vi "ADS-B.vi"() -> ()   [LabVIEW 2020, in "rtlsdr.lvlib"]
uses:
  rtlsdr.lvlib
panel:
  out "second subarray":u8[](array[numeric]) format="%08x"
  out "appended array 2":u8[][](array[numeric]) format="%08x"
  out "substring":string
  out "concatenated string":string
  out "Sample Buffer":u8[](array[numeric])
  in  "stop":bool
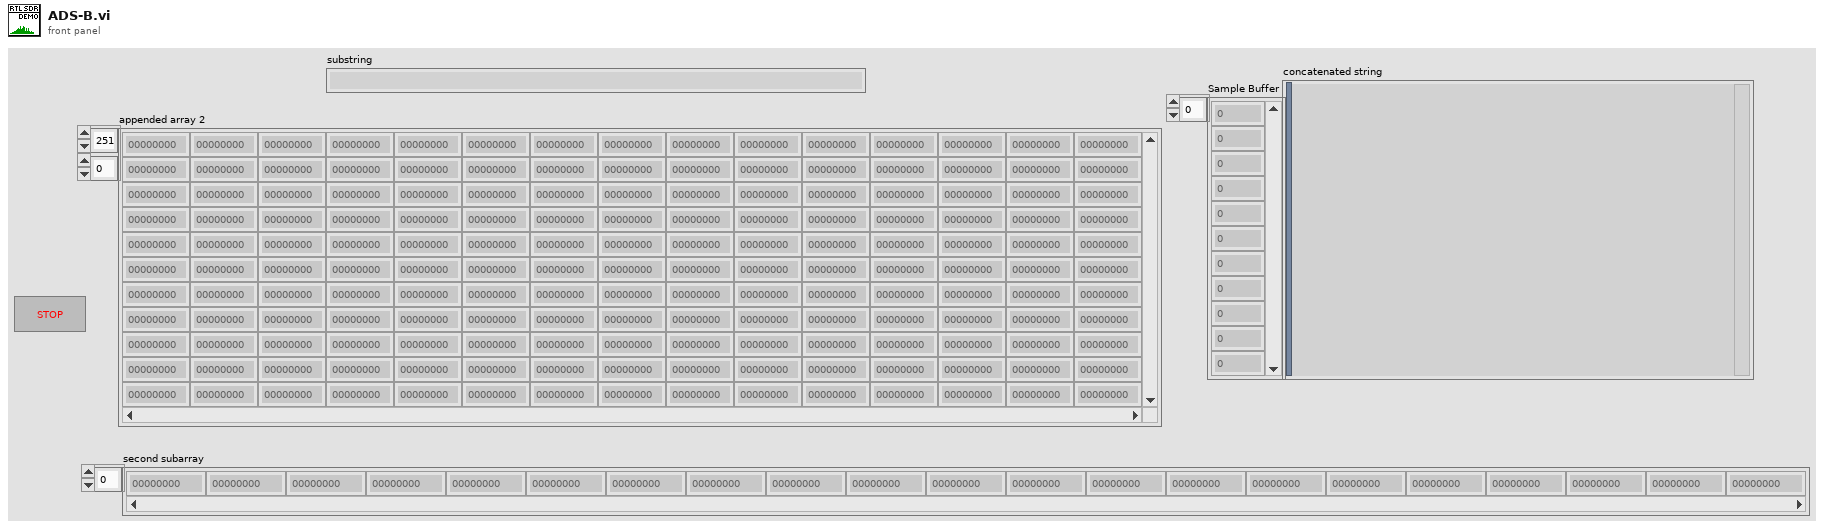
[diagram p1: front panel]
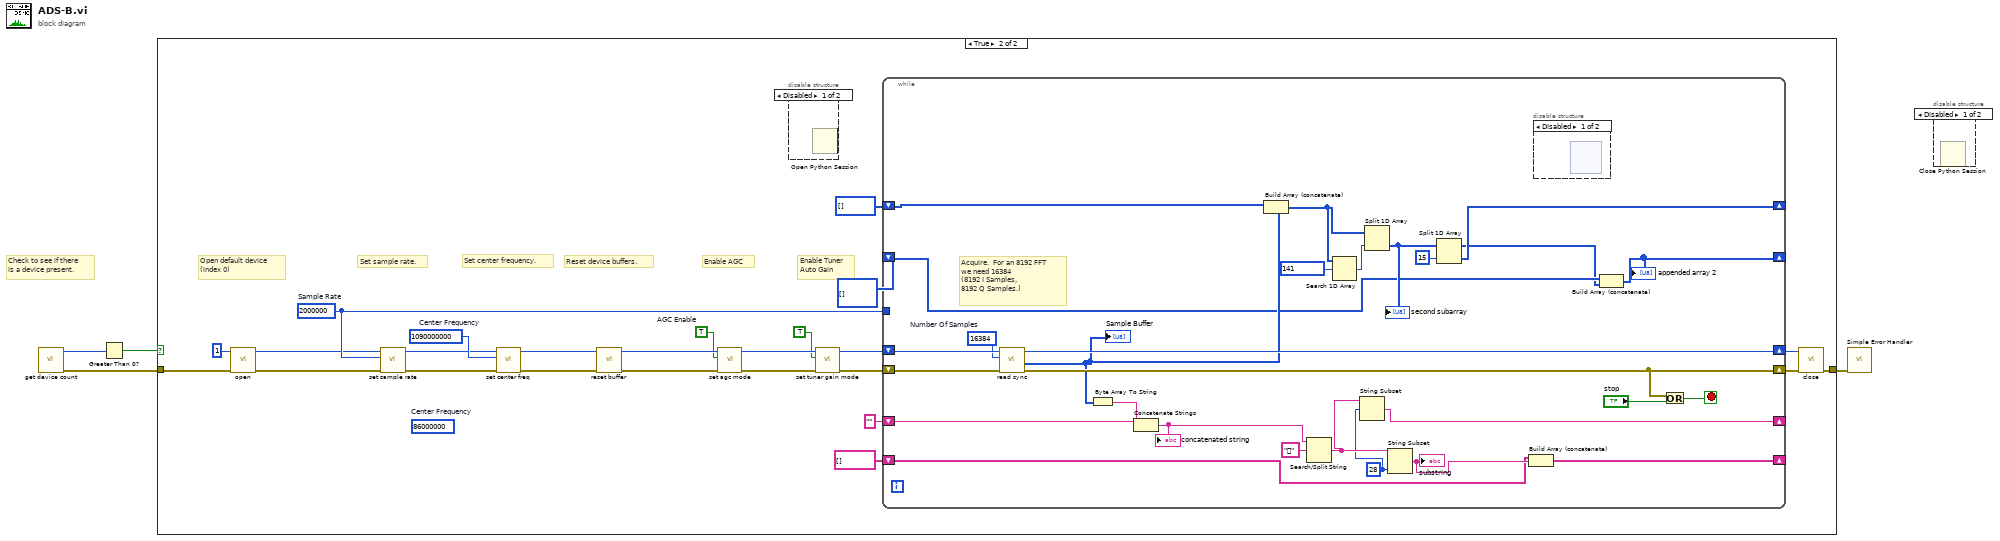
[diagram p0: block diagram]
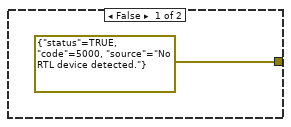
[diagram p3: hidden frame]
diagram:
  # "Check to see if there\nis a device present."
  n1 = call "get device count.vi"() -> ("error out"=w3:errorcluster, "Device Count"=w2:u32)  [unwired: 10 in]
  n2 = Greater Than 0?(x=w2) -> (x > 0?=w1:bool)
  n3 = case shown="True" w1 {
    tunnel: [errorcluster {"status"=TRUE, "code"=5000, "source"="No RTL device detected."} ("error out") w13] -> w4
    tunnel: w3 -> [_ w12]
    frame False {
    }
    frame True {
      (unwired) u32 86000000  # Center Frequency
      w16 = u32 1090000000  # Center Frequency
      w22 = TRUE  # AGC Enable
      w27 = u32 2000000  # Sample Rate
      # "Enable Tuner\nAuto Gain"
      # "Enable AGC"
      # "Reset device buffers."
      # "Set center frequency."
      # "Set sample rate."
      # "Open default device\n(index 0)"
      n4 = call "open.vi"("error in (no error)"=w12, "Device Index"=u32 1 ("index")) -> ("error out"=w17:errorcluster, "DeviceRefnum Out"=w18:u64)  [unwired: 6 in]
      n5 = call "set sample rate.vi"("error in (no error)"=w17, "Sample Rate"=w27, "DeviceRefnum"=w18) -> ("error out"=w15:errorcluster, "DeviceRefnum Out"=w14:u64)  [unwired: 6 in, 1 out]
      n6 = call "set center freq.vi"("error in (no error)"=w15, "Center Frequency"=w16, "DeviceRefnum"=w14) -> ("error out"=w20:errorcluster, "DeviceRefnum Out"=w19:u64)  [unwired: 6 in, 1 out]
      n7 = call "reset buffer.vi"("error in (no error)"=w20, "DeviceRefnum"=w19) -> ("error out"=w26:errorcluster, "DeviceRefnum Out"=w24:u64)  [unwired: 7 in, 1 out]
      n8 = call "set agc mode.vi"("error in (no error)"=w26, "AGC Enable"=w22, "DeviceRefnum"=w24) -> ("error out"=w25:errorcluster, "DeviceRefnum Out"=w23:u64)  [unwired: 6 in, 1 out]
      n9 = disable-structure shown="Disabled" {
        frame Disabled {
          n10 = Open Python Session() -> ()  [unwired: 3 in, 2 out]
        }
        frame Enabled {
        }
      }
      n11 = call "set tuner gain mode.vi"("error in (no error)"=w25, "AutoGain"=TRUE, "DeviceRefnum"=w23) -> ("error out"=w10:errorcluster, "DeviceRefnum Out"=w11:u64)  [unwired: 6 in, 1 out]
      n12 = while {
        tunnel: w27 -> [_]
        shift-right: [w52] -> w28
        shift-left: w11 -> [w58]
        shift-right: [w53] -> w29
        shift-left: w10 -> [w57]
        shift-right: [w45] -> _
        shift-left: "" -> [w50]
        shift-right: [w43] -> _
        shift-left: string[] [] -> [w42]
        shift-right: [w32] -> _
        shift-left: u8[] [] -> [w40]
        shift-right: [w33] -> _
        shift-left: u8[][] [] -> [w34]
        stop <- w54 stop-if-true
        w46 = 28 ("length (rest)")
        w56 = 16384  # Number Of Samples
        # "Acquire.  For an 8192 FFT\nwe need 16384 \n(8192 I Samples,\n8192 Q Samples.)"
        n13 = call "read sync.vi"("error in (no error)"=w57, "Number Of Samples"=w56, "DeviceRefnum"=w58) -> ("error out"=w53:errorcluster, "Sample Buffer"=w41:u8[], "DeviceRefnum Out"=w52:u64)  [unwired: 5 in, 1 out]
        "Sample Buffer" <- w41
        n14 = Byte Array To String(unsigned byte array=w41) -> (string=w51:string)
        n15 = Concatenate Strings(w50, w51) -> (w49:string)
        "concatenated string" <- w49
        n16 = Build Array (concatenate)(w40, w41) -> (w39:u8[])
        n17 = Search/Split String(string=w49, search string/char (-)="") -> (match + rest of string=w47:string)  [unwired: 1 in, 2 out]
        n18 = Search 1D Array(1D array=w39, element=u8 141) -> (index of element=w37:i32)  [unwired: 1 in]
        n19 = String Subset(string=w47, offset (0)=w46) -> (substring=w45:string)  [unwired: 1 in]
        n20 = Split 1D Array(array=w39, index=w37) -> (second subarray=w36:u8[])  [unwired: 1 out]
        "second subarray" <- w36
        n21 = String Subset(string=w47, length (rest)=w46) -> (substring=w44:string)  [unwired: 1 in]
        "substring" <- w44
        n22 = Split 1D Array(array=w36, index=15) -> (first subarray=w31:u8[], second subarray=w32:u8[])
        n23 = Build Array (concatenate)(w42, w44) -> (w43:string[])
        n24 = disable-structure shown="Disabled" {
          frame Disabled {
            n25 = node() -> ()  [unwired: 6 in, 4 out]
          }
          frame Enabled {
          }
        }
        n26 = Build Array (concatenate)(w34, w31) -> (w33:u8[][])
        "appended array 2" <- w33
        n27 = Or(x=w53, y="stop") -> (x .or. y?=w54:bool)
      }
      n28 = call "close.vi"("error in (no error)"=w29, "DeviceRefnum"=w28) -> ("error out"=w13:errorcluster)  [unwired: 8 in, 1 out]
    }
  }
  n29 = call <vilib>:"Simple Error Handler.vi"("error in (no error)"=w4) -> ()  [unwired: 4 in, 5 out]
  n30 = disable-structure shown="Disabled" {
    frame Disabled {
      n31 = Close Python Session() -> ()  [unwired: 2 in, 1 out]
    }
    frame Enabled {
    }
  }
